vi "PythonTest.vi"() -> ()   [LabVIEW 2012]
panel:
  out "error out":errorcluster
  out "standard output":string
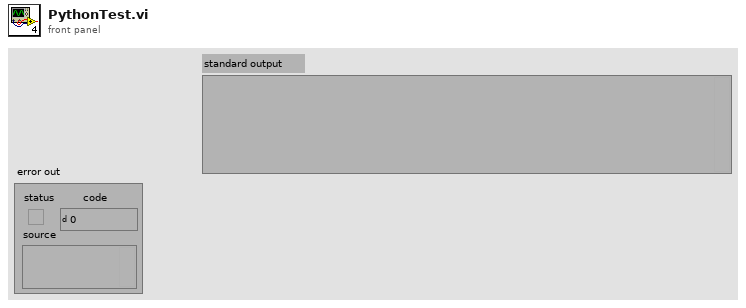
[diagram p1: front panel]
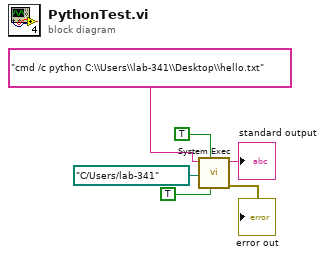
[diagram p0: block diagram]
diagram:
  n1 = call <vilib>:"System Exec.vi"("run minimized? (F)"=TRUE, "wait until completion? (T)"=TRUE, "working directory"=path "C:/Users/lab-341", "command line"="cmd /c python C:\\Users\\lab-341\\Desktop\\hello.txt") -> ("error out"=→"error out":errorcluster, "standard output"=→"standard output":string)  [unwired: 4 in, 2 out]
